vi "ex6_switch case.vi"() -> ()   [LabVIEW 2018]
panel:
  in  "Numeric 2":dbl
  out "Waveform Graph":dbl[](graph)
  out "Waveform Chart":dbl(graph)
  out "Numeric":dbl
  in  "stop":bool
  in  "Knob":dbl(knob) scale=0.2..200.0
  out "Thermometer":dbl(slide) scale=0.0..100.0
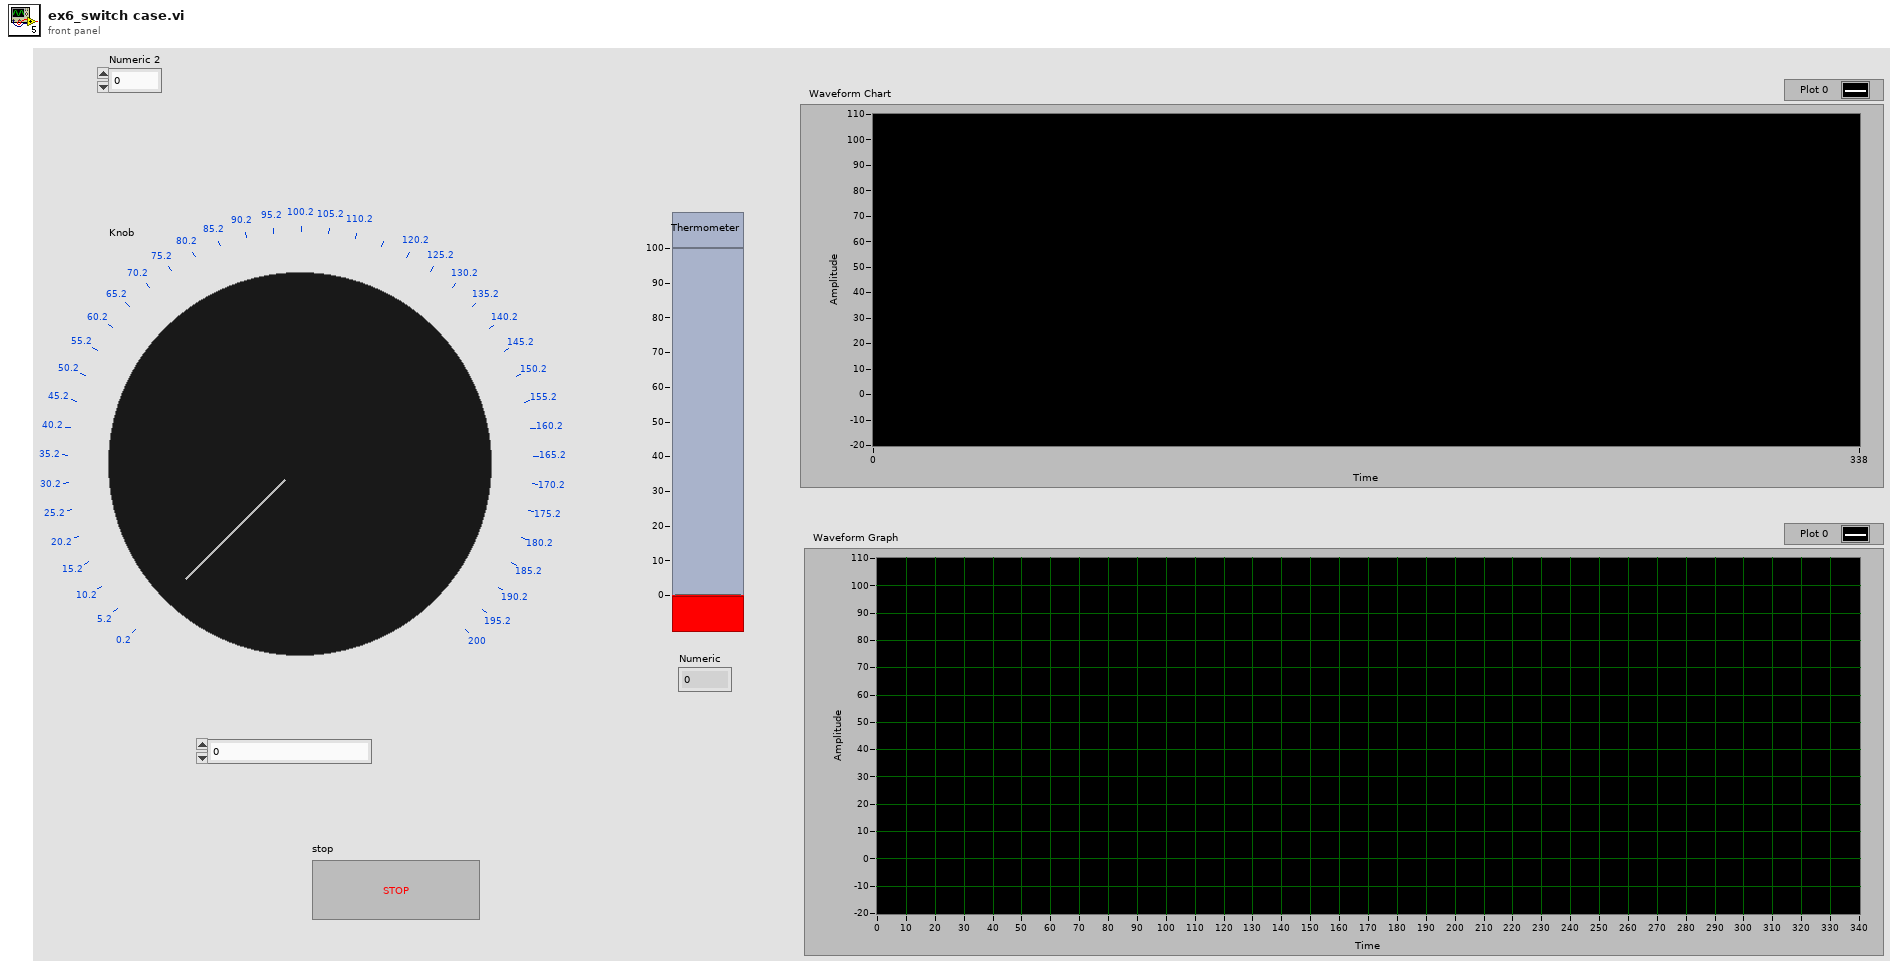
[diagram p1: front panel]
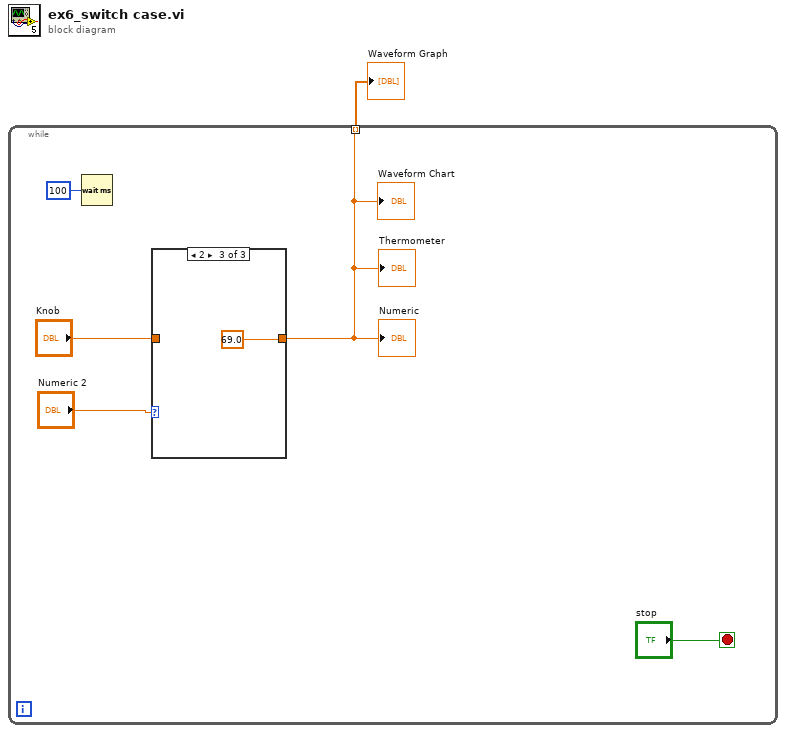
[diagram p0: block diagram]
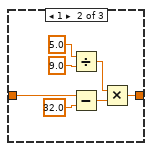
[diagram p3: hidden frame]
diagram:
  n1 = while {
    tunnel: [w3] -> w1 mode=indexing
    stop <- "stop" stop-if-true
    n2 = Wait (ms)(milliseconds to wait=100) -> ()  [unwired: 1 out]
    n3 = case shown="2" "Numeric 2" {
      tunnel: "Knob" -> [w7 w11 _]
      tunnel: [w7 w8 69.0] -> w3
      frame 0, Default {
      }
      frame 1 {
        n4 = Divide(x=5.0, y=9.0) -> (x/y=w10:dbl)
        n5 = Subtract(x=w11, y=32.0) -> (x-y=w9:dbl)
        n6 = Multiply(x=w10, y=w9) -> (x*y=w8:dbl)
      }
      frame 2 {
      }
    }
    "Thermometer" <- w3
    "Numeric" <- w3
    "Waveform Chart" <- w3
  }
  "Waveform Graph" <- w1
